vi "ecg_ncs_v2b.vi"() -> ()   [LabVIEW 2016]
uses:
  <instrlib>/niUSRP/niUSRP Timestamp.ctl
  C:/Program Files/National Instruments/LabVIEW 2016/examples/Instrument IO/Serial/support/Serial - Settings.ctl
  <vilib>/Analysis/coordinate.llb/Wrap Angle (array).vi
  <instrlib>/niUSRP/niUSRP Configure Time Start Trigger.vi
  <vilib>/Instr/_visa.llb/VISA Configure Serial Port (Instr).vi
  <vilib>/Analysis/3filter.llb/Butterworth Filter (DBL).vi
  <instrlib>/niUSRP/niUSRP Write Tx Data (2D CDB).vi
  <instrlib>/niUSRP/niUSRP Fetch Rx Data (2D CDB).vi
  <vilib>/measure/NI_MABase.lvlib
  <vilib>/Analysis/NI_AALBase.lvlib
  <vilib>/Analysis/NI_AALPro.lvlib
  <vilib>/Analysis/NI_AAL_Angle.lvlib
panel:
  out "Array":cdb[][](array[numeric])
  out "size(s) 4":i32[](array[numeric])
  out "timed out?":bool
  out "#sample":i32
  in  "timeout in ms (-1) 2":i32=-1
  in  "timeout in ms (-1)":i32=-1
  out "size(s) 3":i32
  out "size(s) 2":i32=10
  out "Serial Settings: \n#Bytes at Serial Port":u32
  in  "Stop":bool
  out "Poor Sensor Quality: \nSensor off":bool=TRUE
  out "Poor Sensor Quality: \nSensor on":bool
  out "Heart Rate 2":u16[](array[numeric])=[73]
  out "Stop Loop":bool
  out "Loop index":i32=16
  out "size(s)":i32=123
  in  "Read Count":u32=800
  out "return count":u32
  in  "Serial Settings":T1={"baud rate"=57600, "data bits"=8, "parity"=enum."None", "stop bits"=10, "flow control"=0} {"flow control" items=["None"=0, "XON/XOFF"=1, "RTS/CTS"=2, "DTR/DSR"=4]; "stop bits" items=["1.0"=10, "1.5"=15, "2.0"=20]; "data bits" min=5 max=8 step=1; "baud rate" items=["75"=75, "110"=110, "134"=134, "150"=150, "300"=300, "600"=600, "1200"=1200, "1800"=1800, "2400"=2400, "4800"=4800, "7200"=7200, "9600"=9600, "14400"=14400, "19200"=19200, "28800"=28800, "38400"=38400, "56000"=56000, "57600"=57600, "115200"=115200, "128000"=128000, "230400"=230400]}
  in  "VISA resource name":refnum<visa-resource-name>="bmd101"
  in  "?":enum32{"ECG", "Heart Rate"}(tab)
  out "?":i16(graph)=131
  out "?":u8[](graph)=[73]
  in  "File Name":string="Test"
  in  "order1":i32=5
  in  "Path":path=path "D:/Research/SummerFall17Spring18/CnC/NCS/EcgNcsCorrelation"
  in  "Low-Pass Freq":dbl=200.0 format="%#_13g"
  in  "Sampling Rate":i32=500
  out "Gain":dbl=-15.0
  out "Bandwidth":dbl=56000000.0
  out "Coerced Carrier Frequency":dbl=2000000000.0 format="%#.17g"
  out "Coerced Tx IQ rate":dbl=1000000.0
  out "Coerced Rx IQ rate":dbl=1000000.0
  out "error IO":errorcluster={"status"=FALSE, "code"=-1074118647, "source"=""}
  in  "Rx Number of Samples":i32=20000
  in  "Tab Control 2":enum32{"NI-294x/295x", "NI-2900/2901"}(tab)=enum."NI-2900/2901"
  in  "channel 0 carrier\n frequency [Hz]":dbl=2000000000.0 format="%#_6p"
  in  "Rx carrier frequency [Hz]":dbl=2000000000.0 format="%#_6p"
  in  "Tx carrier frequency [Hz]":dbl=1000000000.0 format="%#_6p"
  in  "Start Trigger Time":T2={"whole seconds"=1, "fractional seconds"=0.0}
  out "Tx Active Antenna":string="TX1"
  in  "Tab Control":T3(tab)
  out "NCS tag Amp":dbl[](graph)=[0.012547740464413999, 0.012546996275393813, 0.012546251124152991, 0.012545505011287303, 0.012544757937393139, 0.012544009903067494, 0.012543260908907984, 0.012542510955512811, 0.012541760043480784, 0.012541008173411305]
  out "NCS tag Phase":dbl[](graph)=[-1.392700873477184e-06, -1.383717662048323e-06, -1.3747392404395601e-06, -1.365765619105003e-06, -1.3567968084830664e-06, -1.3478328189964664e-06, -1.3388736610522184e-06, -1.3299193450416306e-06, -1.3209698813403015e-06, -1.3120252803081151e-06]
  out "IQ":dbl[][](graph)=[[-0.008331551052877154], [0.0]]
  out "Tag Amp":dbl[](graph)=[0.008331551052877154]
  out "Tag Phase":dbl[](graph)=[337.4998459209021]
  out "Tx Waveform Graph":waveform(dbl)[](graph)
  in  "Channel 0\nTone Amplitude":dbl=0.707 step=0.05 format="%#.6g"
  in  "Channel 0 \nTone Frequency":dbl=5000.0 format="%#_6p"
  in  "Waveform Size":dbl=1000.0
  in  "Rx Active Antenna":string="RX2"
  in  "Device Name":refnum<k15>="MyB200"
  in  "Tx Gain":dbl=28.0 format="%#_6f"
  in  "Tx IQ Rate":dbl=1000000.0 format="%#_6p"
  in  "Rx Gain":dbl=32.0 format="%#_6f"
  in  "Rx IQ Rate":dbl=1000000.0 format="%#_6p"
  # "Rx Settings"
  # "Tx Settings"
  # "Note that on the NI-2900 and NI-2901, both Rx channels share an LO and both Tx channels share an LO. However, on the NI-294x/295x devices, Rx and Tx of channel 0 share an LO and Rx and Tx of channel 1 share an LO."
  # "This Tx graph should always have end and start tied up since this is being sent in a loop continuously. Otherwise phase jumps will be noticed."
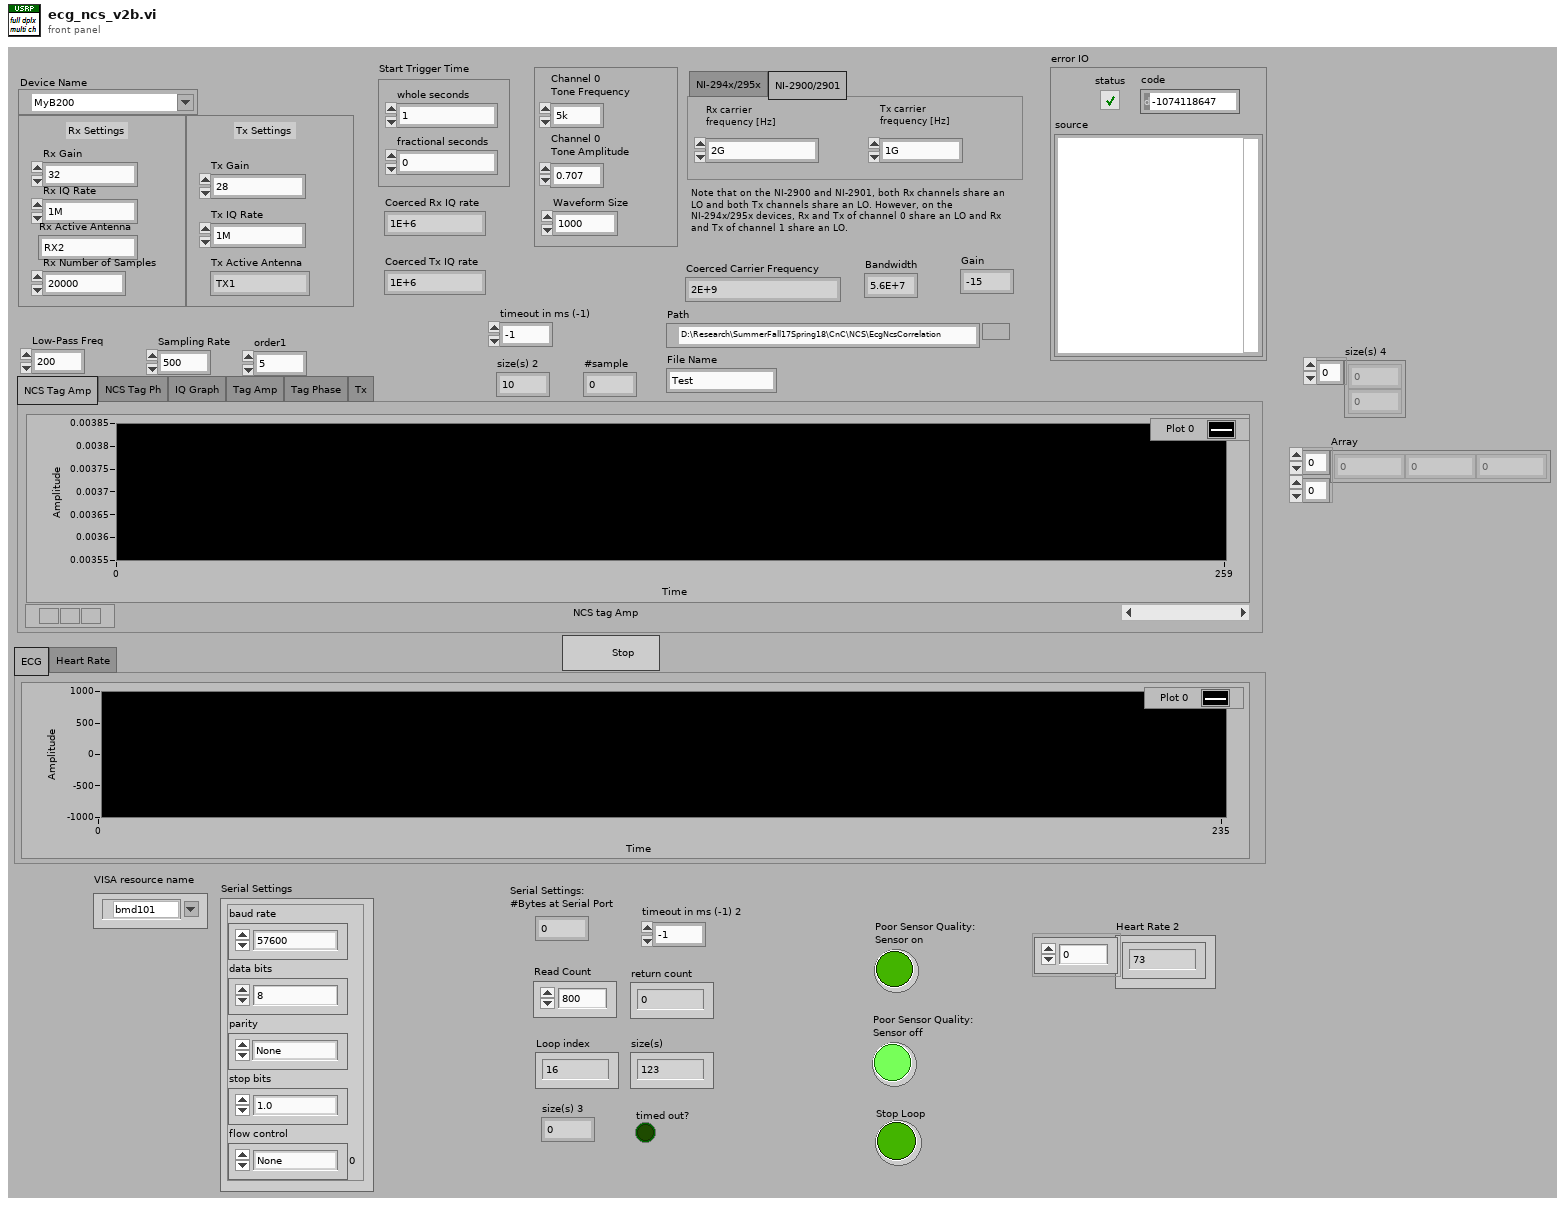
[diagram p1: front panel]
types:
  T1 = typedef "Serial - Settings.ctl" = cluster{"baud rate":u32, "data bits":u16, "parity":enum16{"None", "Odd", "Even", "Mark", "Space"}, "stop bits":u16, "flow control":u16}
  T2 = typedef "niUSRP Timestamp.ctl" = cluster{"whole seconds":u64, "fractional seconds":dbl}
  T3 = enum32{"NCS Tag Amp", "NCS Tag Ph", "IQ Graph", "Tag Amp", "Tag Phase", "Tx"}
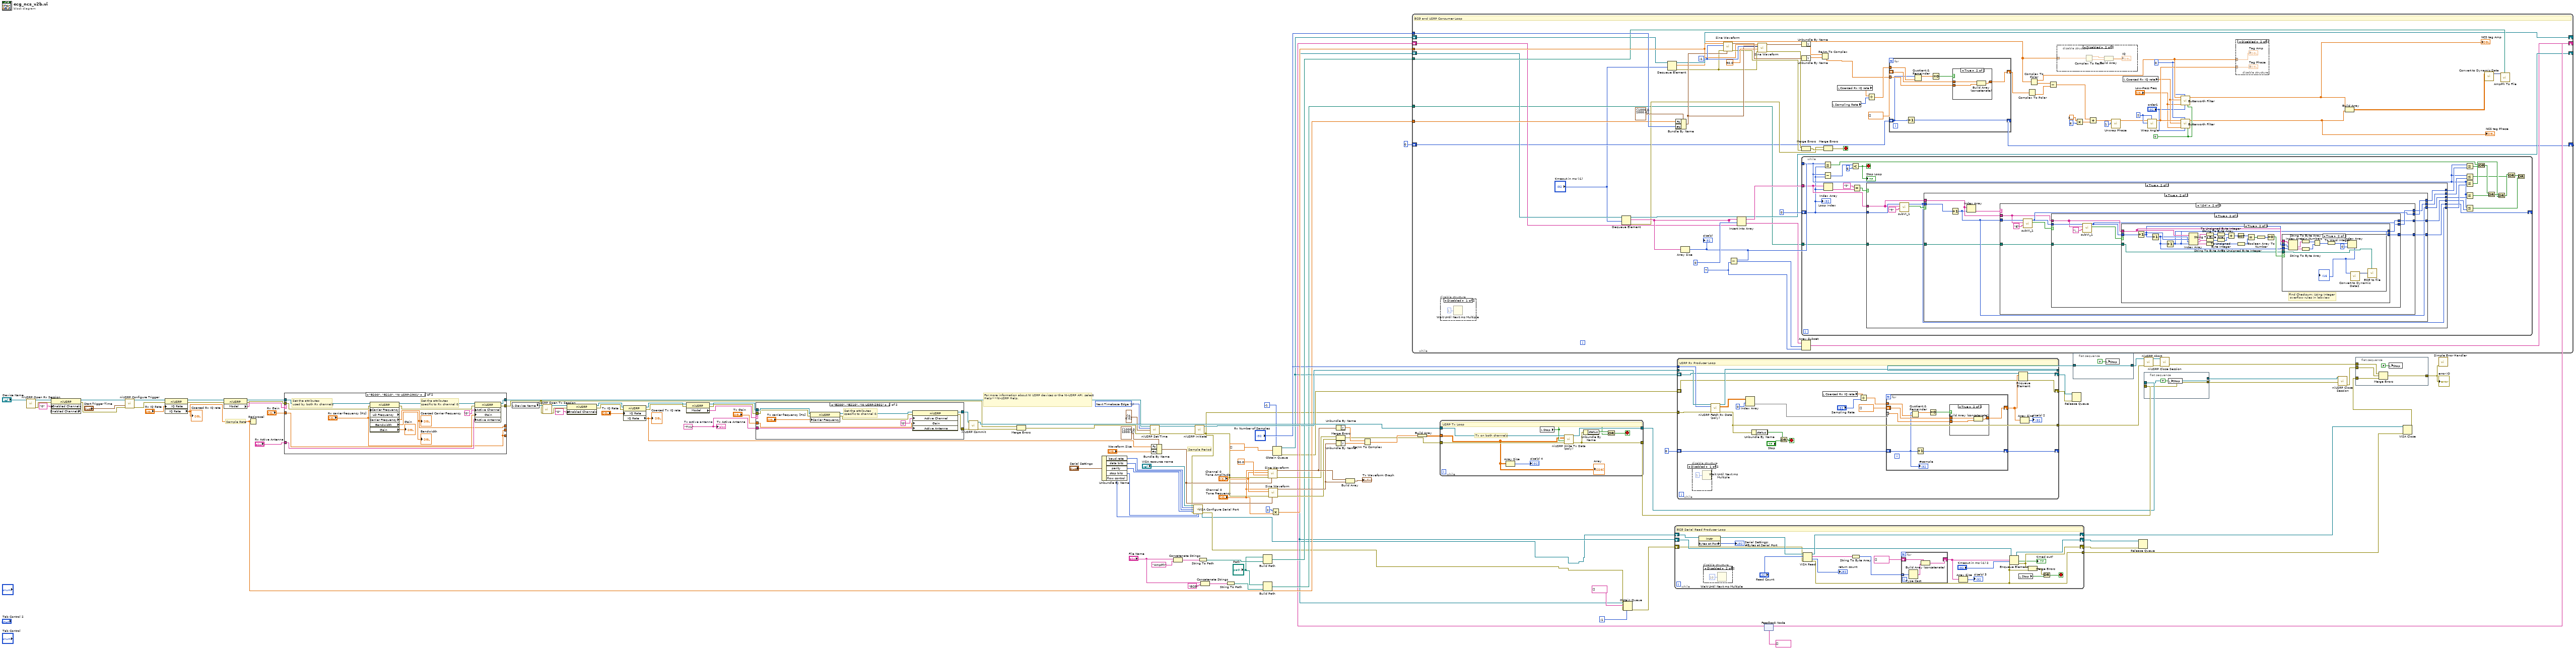
[diagram p0: block diagram]
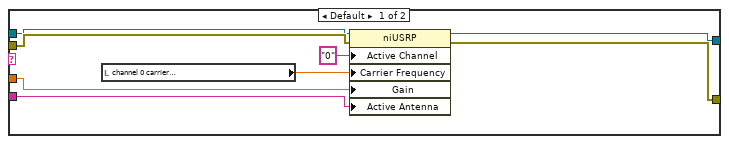
[diagram p5: hidden frame]
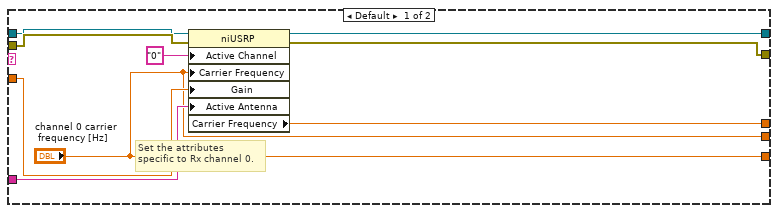
[diagram p6: hidden frame]
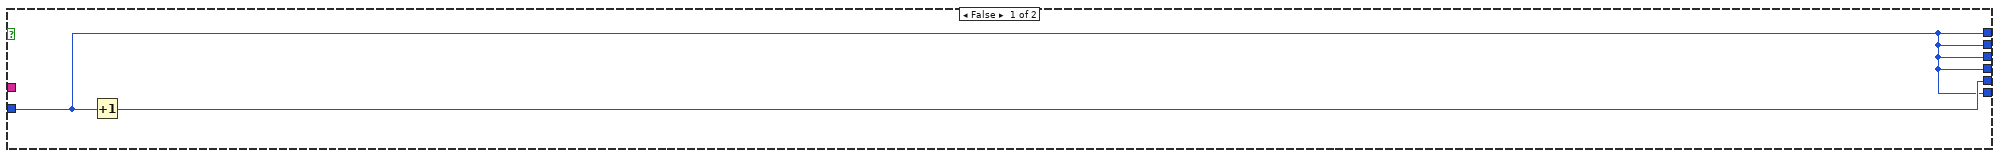
[diagram p9: hidden frame]
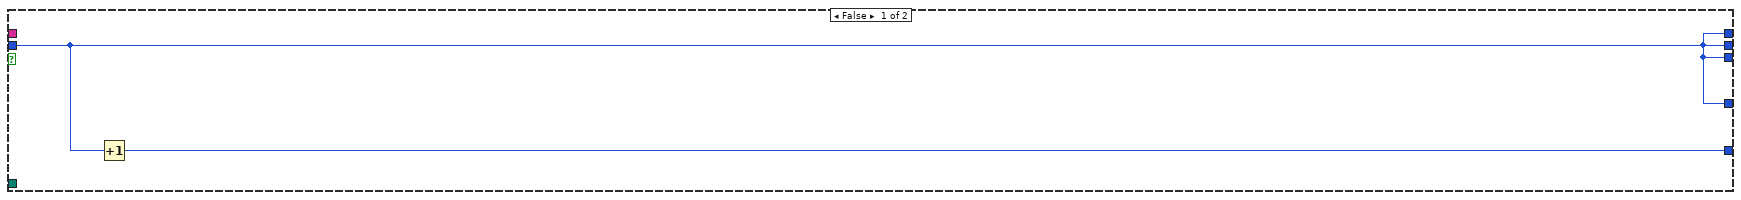
[diagram p10: hidden frame]
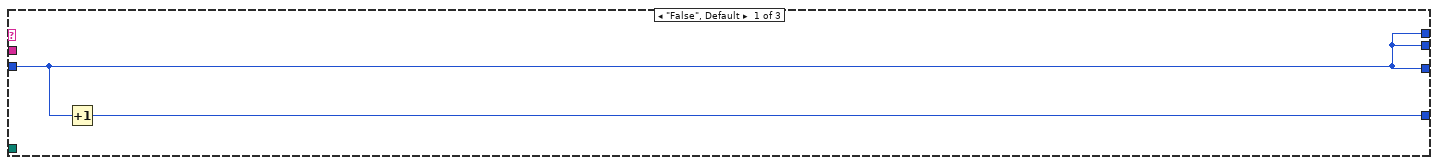
[diagram p11: hidden frame]
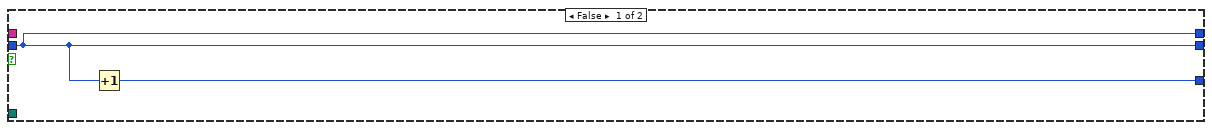
[diagram p12: hidden frame]
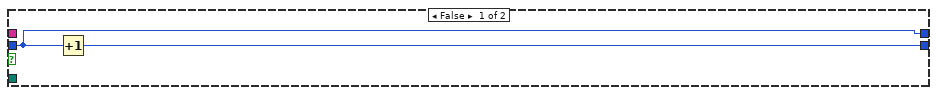
[diagram p13: hidden frame]
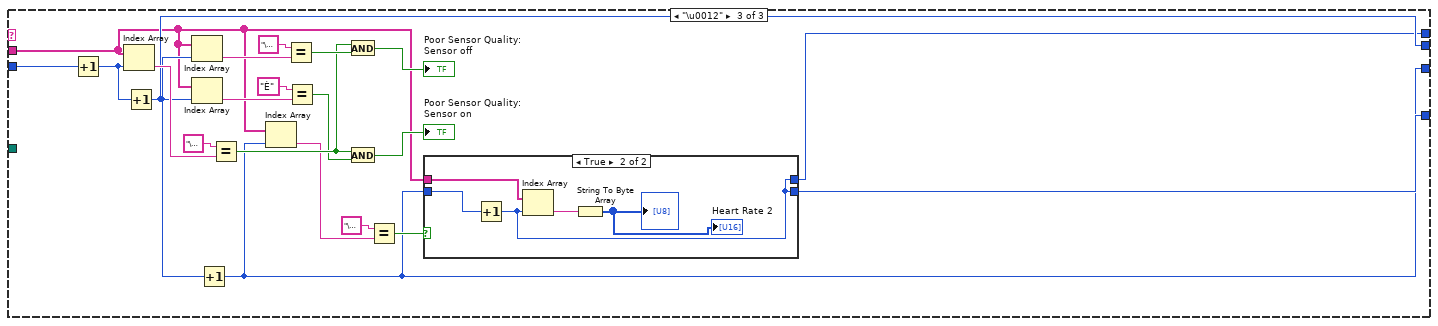
[diagram p15: hidden frame]
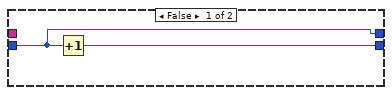
[diagram p16: hidden frame]
diagram:
  w91 = 1 items=["Now", "Next Timebase Edge"] ("apply timestamp")
  w60 = "TX1"  # Tx active antenna
  # "Sample Rate"
  # "Sample Period"
  # "For more information about NI USRP devices or the NI-USRP API, select Help>>NI-USRP Help."
  n1 = call <instrlib>:"niUSRP Open Rx Session.vi"("device names"="Device Name") -> ("session handle out"=w90:refnum<k15>, "error out"=w89:errorcluster)  [unwired: 13 in]
  n2 = property class="niUSRP" props=["Enabled Channels", "Enabled Channels"](reference=w90, error in=w89, "Enabled Channels"="0" ("Configuration:Enabled Channels")) -> (reference out=w88:refnum<k15>, error out=w87:errorcluster)  [unwired: 1 out]
  n3 = call-poly <instrlib>:"niUSRP Configure Trigger.vi"("session handle"=w88, "start trigger time"="Start Trigger Time", "error in (no error)"=w87) -> ("session handle out"=w84:refnum<k15>, "error out"=w83:errorcluster)  [unwired: 11 in]
  n4 = property class="niUSRP"(reference=w84, error in=w83, "IQ Rate"="Rx IQ Rate") -> (reference out=w80:refnum<k15>, error out=w81:errorcluster, "IQ Rate"=w19:dbl)
  "Coerced Rx IQ rate" <- w19
  n5 = property class="niUSRP"(reference=w80, error in=w81) -> (reference out=w75:refnum<k15>, error out=w76:errorcluster, "Model"=w77:string)
  n6 = Reciprocal(x=w19) -> ()  [unwired: 1 out]
  n7 = case shown="\"B200\", \"B210\", \"NI USRP-2901\"" w77 {
    tunnel: w76 -> [w124 w134]
    tunnel: w75 -> [w123 w135]
    tunnel: [w120 w131] -> w79
    tunnel: [w119 w130] -> w78
    tunnel: "Rx Gain" -> [w122 w137]
    tunnel: "Rx Active Antenna" -> [w121 w136]
    tunnel: [w117 w126] -> _
    tunnel: ["channel 0 carrier\n frequency [Hz]" "Rx carrier frequency [Hz]"] -> _
    tunnel: ["channel 0 carrier\n frequency [Hz]" "Rx carrier frequency [Hz]"] -> _
    frame Default {
      # "Set the attributes \nspecific to Rx channel 0."
      n8 = property class="niUSRP"(reference=w123, error in=w124, "Active Channel"="0", "Carrier Frequency"="channel 0 carrier\n frequency [Hz]", "Gain"=w122, "Active Antenna"=w121) -> (reference out=w120:refnum<k15>, error out=w119:errorcluster, "Carrier Frequency"=w117:dbl)
    }
    frame "B200", "B210", "NI USRP-2901" {
      # "Set the attributes \nused by both Rx channels"
      # "Set the attributes \nspecific to Rx channel 0."
      n9 = property class="niUSRP" props=["Carrier Frequency", "LO Frequency", "Carrier Frequency", "Bandwidth", "Gain"](reference=w135, error in=w134, "Carrier Frequency"="Rx carrier frequency [Hz]") -> (reference out=w133:refnum<k15>, error out=w132:errorcluster, "Carrier Frequency"=w126:dbl, "Bandwidth"=→"Bandwidth":dbl, "Gain"=→"Gain":dbl)  [unwired: 1 out]
      "Coerced Carrier Frequency" <- w126
      n10 = property class="niUSRP"(reference=w133, error in=w132, "Active Channel"="0", "Gain"=w137, "Active Antenna"=w136) -> (reference out=w131:refnum<k15>, error out=w130:errorcluster)
    }
  }
  n11 = local read "Device Name"() -> (w111:refnum<k15>)
  n12 = call <instrlib>:"niUSRP Open Tx Session.vi"("device names"=w111, "error in (no error)"=w78) -> ("session handle out"=w86:refnum<k15>, "error out"=w85:errorcluster)  [unwired: 12 in]
  n13 = property class="niUSRP"(reference=w86, error in=w85, "Enabled Channels"="0" ("Configuration:Enabled Channels")) -> (reference out=w72:refnum<k15>, error out=w71:errorcluster)
  n14 = property class="niUSRP"(reference=w72, error in=w71, "IQ Rate"="Tx IQ Rate") -> (reference out=w66:refnum<k15>, error out=w67:errorcluster, "IQ Rate"=w64:dbl)
  "Coerced Tx IQ rate" <- w64
  n15 = property class="niUSRP"(reference=w66, error in=w67) -> (reference out=w68:refnum<k15>, error out=w69:errorcluster, "Model"=w65:string)
  n16 = case shown="\"B200\", \"B210\", \"NI USRP-2901\"" w65 {
    tunnel: "Tx Gain" -> [w146 w156]
    tunnel: w60 -> [w144 w154]
    tunnel: [w140 w148] -> w62
    tunnel: [w139 w147] -> w63
    tunnel: w69 -> [w143 w150]
    tunnel: w68 -> [w142 w153]
    frame Default {
      n17 = local read "channel 0 carrier\n frequency [Hz]"() -> (w141:dbl)
      n18 = property class="niUSRP"(reference=w142, error in=w143, "Active Channel"="0", "Carrier Frequency"=w141, "Gain"=w146, "Active Antenna"=w144) -> (reference out=w140:refnum<k15>, error out=w139:errorcluster)
    }
    frame "B200", "B210", "NI USRP-2901" {
      # "Set the attributes \nspecific to channel 0."
      n19 = property class="niUSRP"(reference=w153, error in=w150, "Carrier Frequency"="Tx carrier frequency [Hz]") -> (reference out=w152:refnum<k15>, error out=w151:errorcluster)
      n20 = property class="niUSRP"(reference=w152, error in=w151, "Active Channel"="0", "Gain"=w156, "Active Antenna"=w154) -> (reference out=w148:refnum<k15>, error out=w147:errorcluster)
    }
  }
  n21 = call <instrlib>:"niUSRP Commit.vi"("session handle"=w62, "error in (no error)"=w63) -> ("session handle out"=w113:refnum<k15>, "error out"=w114:errorcluster)  [unwired: 12 in]
  n22 = Merge Errors(w78, w114) -> (w93:errorcluster)
  n23 = Unbundle By Name("Serial Settings") -> ("baud rate"=w26:u32, "data bits"=w27:u16, "parity"=w28:enum16{"None", "Odd", "Even", "Mark", "Space"}, "stop bits"=w29:u16, "flow control"=w30:u16)
  n24 = call <instrlib>:"niUSRP Set Time.vi"("session handle"=w79, "apply timestamp"=w91, "timestamp"=T2 {"whole seconds"=0, "fractional seconds"=0.0}, "error in (no error)"=w93) -> ("session handle out"=w95:refnum<k15>, "error out"=w94:errorcluster)  [unwired: 10 in]
  n25 = Bundle By Name(cluster=cluster{"Fs":dbl, "#s":dbl} {"Fs"=1000.0, "#s"=1000.0} ("sampling info"), "Fs"=w64, "#s"="Waveform Size") -> (w97:cluster{"Fs":dbl, "#s":dbl})
  n26 = Concatenate Strings("File Name", "AmpPh") -> (w44:string)
  n27 = call <instrlib>:"niUSRP Initiate.vi"("session handle"=w95, "error in (no error)"=w94) -> ("session handle out"=w22:refnum<k15>, "error out"=w1:errorcluster)  [unwired: 12 in]
  n28 = call-poly "VISA Configure Serial Port"("VISA resource name"="VISA resource name", "baud rate (9600)"=w26, "data bits (8)"=w27, "parity (0:none)"=w28, "error in (no error)"=w1, "stop bits (10: 1 bit)"=w29, "flow control (0:none)"=w30) -> ("VISA resource name out"=w2:refnum<visa-resource-name>, "error out"=w3:errorcluster)  [unwired: 3 in, 4 out]
  n29 = String To Path(string=w44) -> (path=w43:path)
  n30 = Concatenate Strings("File Name", "ECG") -> (w38:string)
  n31 = String To Path(string=w38) -> (path=w37:path)
  n32 = Build Path(base path="Path", name or relative path=w43) -> (appended path=w46:path)
  n33 = Build Path(base path="Path", name or relative path=w37) -> (appended path=w14:path)
  n34 = call <vilib>:"Sine Waveform.vi"("sampling info"=w97, "error in (no error)"=w1, "phase"=90.0, "amplitude"="Channel 0\nTone Amplitude", "frequency"="Channel 0 \nTone Frequency") -> ("error out"=w58:errorcluster, "signal out"=w105:waveform(dbl))  [unwired: 5 in]
  n35 = call <vilib>:"Sine Waveform.vi"("sampling info"=w97, "error in (no error)"=w1, "amplitude"="Channel 0\nTone Amplitude", "frequency"="Channel 0 \nTone Frequency") -> ("error out"=w59:errorcluster, "signal out"=w106:waveform(dbl))  [unwired: 6 in]
  n36 = Multiply(x=2, y="Channel 0 \nTone Frequency") -> (x*y=w47:dbl)
  n37 = Obtain Queue(max queue size (-1, unlimited)=-1, element data type=dbl[] []) -> (queue out=w16:refnum<queue>, error out=w5:errorcluster)  [unwired: 3 in, 1 out]
  n38 = Unbundle By Name(w105) -> ("Y"=w104:dbl[])
  n39 = Merge Errors(w58, w59) -> (w57:errorcluster)
  n40 = Unbundle By Name(w106) -> ("Y"=w103:dbl[])
  n41 = Build Array(w105, w106) -> (→"Tx Waveform Graph":waveform(dbl)[])
  n42 = Re/Im To Complex(1:w103, 2:w104) -> (0:w99:cdb[])
  n43 = Build Array(w99) -> (w98:cdb[][])
  n44 = while {
    tunnel: w113 -> [w165]
    tunnel: w57 -> [w164]
    tunnel: [w162] -> w56
    tunnel: [w160] -> w52
    tunnel: w98 -> [w158]
    stop <- w161 stop-if-true
    # "Tx on both channels"
    # "USRP Tx Loop"
    n45 = Array Size(array=w158) -> (size(s)=→"size(s) 4":i32[])
    n46 = local read "Stop"() -> (w159:bool)
    n47 = call-poly <instrlib>:"niUSRP Write Tx Data (poly).vi"("session handle"=w165, "data"=w158, "end of data?"=w159, "error in (no error)"=w164) -> ("session handle out"=w160:refnum<k15>, "error out"=w162:errorcluster)  [unwired: 10 in]
    n48 = Unbundle By Name(w162) -> ("status"=w163:bool)
    n49 = Compound Arithmetic op=OR(w163, w159) -> (w161:bool)
    "Array" <- w158
  }
  n50 = Obtain Queue(max queue size (-1, unlimited)=-1, element data type=string[] [], error in (no error)=w3) -> (queue out=w13:refnum<queue>, error out=w32:errorcluster)  [unwired: 2 in, 1 out]
  n51 = while {
    tunnel: [w166] -> w36
    shift-right: [w180] -> w34
    shift-left: w32 -> [w167]
    shift-right: [w181] -> w33
    shift-left: w13 -> [w182]
    shift-right: [w184] -> w35
    shift-left: w2 -> [w168]
    stop <- w186 stop-if-true
    # "ECG Serial Read Producer Loop"
    n52 = property class="Instr"(reference=w168) -> (reference out=w177:refnum<visa-resource-name>, "Bytes at Port"=→"Serial Settings: \n#Bytes at Serial Port":u32)  [unwired: 1 in, 1 out]
    n53 = disable-structure shown="Disabled" {
      frame Enabled {
      }
      frame Disabled {
        n54 = Wait Until Next ms Multiple(millisecond multiple=u32 10) -> ()  [unwired: 1 out]
      }
    }
    n55 = VISA Read(VISA resource name=w177, byte count="Read Count", error in (no error)=w167) -> (VISA resource name out=w184:refnum<visa-resource-name>, read buffer=w176:string, return count=→"return count":u32, error out=w166:errorcluster)
    n56 = String To Byte Array(string=w176) -> (unsigned byte array=w183:u8[])
    n57 = for {
      tunnel: w183 -> [w191] mode=indexing
      shift-right: [w188] -> w174
      shift-left: string[] [] -> [w189]
      n58 = Type Cast(x=w191) -> (*(type *) &x=w190:string)  [unwired: 1 in]
      n59 = Build Array (concatenate)(w189, w190) -> (w188:string[])
    }
    n60 = Array Size(array=w174) -> (size(s)=→"size(s) 3":i32)
    n61 = Enqueue Element(queue=w182, element=w174, timeout in ms (-1)="timeout in ms (-1) 2", error in (no error)=w166) -> (queue out=w181:refnum<queue>, timed out?=→"timed out?":bool, error out=w180:errorcluster)
    n62 = local read "Stop"() -> (w178:bool)
    n63 = Merge Errors(w180, w166) -> (w179:errorcluster)
    n64 = Or(x=w179, y=w178) -> (x .or. y?=w186:bool)
  }
  n65 = while {
    tunnel: w22 -> [w213]
    tunnel: [w212] -> w21
    tunnel: "Rx Number of Samples" -> [w211]
    tunnel: [w206] -> w15
    shift-right: [w208] -> w17
    shift-left: w16 -> [w209]
    shift-right: [w194] -> _
    shift-left: 0 -> [w195]
    tunnel: w1 -> [w207]
    shift-right: [w193] -> w4
    shift-left: w5 -> [w192]
    stop <- w210 stop-if-true
    # "USRP Rx Producer Loop"
    n66 = disable-structure shown="Disabled" {
      frame Disabled {
        n67 = Wait Until Next ms Multiple(millisecond multiple=u32 1 ("milliseconds to wait")) -> ()  [unwired: 1 out]
      }
      frame Enabled {
      }
    }
    n68 = call-poly <instrlib>:"niUSRP Fetch Rx Data (poly).vi"("session handle"=w213, "number of samples"=w211, "error in (no error)"=w207) -> ("session handle out"=w212:refnum<k15>, "data"=w204:cdb[][], "error out"=w206:errorcluster)  [unwired: 9 in, 1 out]
    n69 = Index Array(array=w204, index (row)=0 ("y")) -> (element=w198:cdb[])  [unwired: 1 in]
    n70 = Unbundle By Name(w206) -> ("status"=w214:bool)
    n71 = Or(x=w214, y="Stop") -> (x .or. y?=w210:bool)
    n72 = local read "Coerced Rx IQ rate"() -> (w202:dbl)
    n73 = Divide(x=w202, y="Sampling Rate") -> (x/y=w200:dbl)
    n74 = for {
      tunnel: w198 -> [w222] mode=indexing
      shift-right: [w220] -> w197
      shift-left: dbl[] [] -> [w221]
      tunnel: w200 -> [w217]
      shift-right: [w215] -> w194
      shift-left: w195 -> [w216]
      n75 = Quotient & Remainder(x=w216, y=w217) -> (x-y*floor(x/y)=w218:dbl)  [unwired: 1 out]
      n76 = Increment(x=w216) -> (x+1=w215:i32)
      n77 = Equal To 0?(x=w218) -> (x = 0?=w219:bool)
      n78 = case shown="True" w219 {
        tunnel: w222 -> [_ w226]
        tunnel: w221 -> [w223 w225]
        tunnel: [w223 w224] -> w220
        frame False {
        }
        frame True {
          n79 = Build Array (concatenate)(w225, w226) -> (w224:cdb[])
        }
      }
      "#sample" <- w216
    }
    n80 = Enqueue Element(queue=w209, element=w197, error in (no error)=w192) -> (queue out=w208:refnum<queue>, error out=w193:errorcluster)  [unwired: 1 in, 1 out]
    n81 = Array Size(array=w197) -> (size(s)=→"size(s) 2":i32)
  }
  n82 = feedback #1(string[] []) -> (w9:string[])
  n83 = while {
    tunnel: "Rx Number of Samples" -> [w288]
    tunnel: w19 -> [w280]
    tunnel: w47 -> [w281]
    tunnel: w46 -> [w279]
    shift-right: [w257] -> _
    shift-left: w16 -> [w258]
    tunnel: w14 -> [w234]
    shift-right: [w249] -> _
    shift-left: w13 -> [w250]
    shift-right: [w246] -> w12
    shift-left: w9 -> [w245]
    shift-right: [w229] -> _
    shift-left: 0 -> [w230]
    stop <- w248 stop-if-true
    w254 = 7
    w268 = 2 ("y")
    w261 = TRUE
    w263 = 0
    w286 = -1
    # "ECG and USRP Consumer Loop"
    n84 = disable-structure shown="Disabled" {
      frame Disabled {
        n85 = Wait Until Next ms Multiple(millisecond multiple=u32 1) -> ()  [unwired: 1 out]
      }
      frame Enabled {
      }
    }
    n86 = Dequeue Element(queue=w250, timeout in ms (-1)="timeout in ms (-1)") -> (queue out=w249:refnum<queue>, element=w247:string[], error out=w242:errorcluster)  [unwired: 1 in, 1 out]
    n87 = Dequeue Element(queue=w258, timeout in ms (-1)="timeout in ms (-1)") -> (queue out=w257:refnum<queue>, element=w241:dbl[], error out=w244:errorcluster)  [unwired: 1 in, 1 out]
    n88 = Bundle By Name(cluster=cluster{"Fs":dbl, "#s":dbl} {"Fs"=1000.0, "#s"=1000.0} ("sampling info"), "Fs"=w280, "#s"=w288) -> (w285:cluster{"Fs":dbl, "#s":dbl})
    n89 = Array Size(array=w247) -> (size(s)=w252:i32)
    "size(s)" <- w252
    n90 = call <vilib>:"Sine Waveform.vi"("sampling info"=w285, "error in (no error)"=w244, "amplitude"=w286, "frequency"=w281) -> ("error out"=w284:errorcluster, "signal out"=w289:waveform(dbl))  [unwired: 6 in]
    n91 = Subtract(x=w252, y=w254) -> (x-y=w253:i32)
    n92 = Insert Into Array(array=w247, index=0, new element=w245) -> (w255:string[])
    n93 = call <vilib>:"Sine Waveform.vi"("sampling info"=w285, "error in (no error)"=w244, "phase"=90.0, "amplitude"=w286, "frequency"=w281) -> ("error out"=w283:errorcluster, "signal out"=w282:waveform(dbl))  [unwired: 5 in]
    n94 = Unbundle By Name(w282) -> ("Y"=w277:dbl[])
    n95 = Unbundle By Name(w289) -> ("Y"=w276:dbl[])
    n96 = Merge Errors(w283, w284) -> (w243:errorcluster)
    n97 = while {
      tunnel: w255 -> [w325]
      shift-right: [w329] -> _
      shift-left: 0 -> [w308]
      tunnel: w252 -> [w309]
      tunnel: w234 -> [w304]
      stop <- w305 stop-if-true
      n98 = Less Or Equal?(x=w309, y=w308) -> (x <= y?=w310:bool)
      n99 = Subtract(x=w309, y=w308) -> (x-y=w307:i32)
      n100 = Index Array(array=w325, index=w308) -> (element=w328:string)
      n101 = Less?(x=w307, y=6) -> (x < y?=w305:bool)
      "Stop Loop" <- w305
      n102 = Equal?(x="ª", y=w328) -> (x = y?=w326:bool)
      n103 = case shown="True" w326 {
        tunnel: w308 -> [w330 w341]
        tunnel: [w331 w339] -> w329
        tunnel: w325 -> [_ w333]
        tunnel: [w330 w338] -> w324
        tunnel: [w330 w337] -> w322
        tunnel: [w330 w336] -> w319
        tunnel: [w330 w335] -> w316
        tunnel: [w330 w334] -> w313
        tunnel: w304 -> [_ w332]
        frame False {
          n104 = Increment(x=w330) -> (x+1=w331:i32)
        }
        frame True {
          n105 = call "subVI_1.vi"("String"="ª", "Array"=w333, "Numeric in"=w341) -> ("Boolean"=w340:bool, "Numeric out"=w338:i32)  [unwired: 7 in]
          n106 = case shown="True" w340 {
            tunnel: w338 -> [w343 w347]
            tunnel: [w344 w353] -> w339
            tunnel: w333 -> [_ w352]
            tunnel: [w343 w348] -> w337
            tunnel: [w343 w351] -> w336
            tunnel: [w343 w350] -> w335
            tunnel: [w343 w349] -> w334
            tunnel: w332 -> [_ w345]
            frame False {
              n107 = Increment(x=w343) -> (x+1=w344:i32)
            }
            frame True {
              n108 = Increment(x=w347) -> (x+1=w348:i32)
              n109 = Index Array(array=w352, index=w348) -> (element=w346:string)
              n110 = case shown="\"\\04\"" w346 {
                tunnel: w348 -> [w354 w361 w429]
                tunnel: [w355 w364 w411] -> w353
                tunnel: w352 -> [_ w357 w413]
                tunnel: [w354 w359 w415] -> w351
                tunnel: [w354 w363 w412] -> w350
                tunnel: [w354 w362 w410] -> w349
                tunnel: w345 -> [_ w356 _]
                frame "False", Default {
                  n111 = Increment(x=w354) -> (x+1=w355:i32)
                }
                frame "\u0004" {
                  n112 = call "subVI_1.vi"("String"="€", "Array"=w357, "Numeric in"=w361) -> ("Boolean"=w358:bool, "Numeric out"=w359:i32)  [unwired: 7 in]
                  n113 = case shown="True" w358 {
                    tunnel: w359 -> [w365 w372]
                    tunnel: [w366 w374] -> w364
                    tunnel: w357 -> [_ w371]
                    tunnel: [w365 w369] -> w363
                    tunnel: [w365 w373] -> w362
                    tunnel: w356 -> [_ w367]
                    frame False {
                      n114 = Increment(x=w365) -> (x+1=w366:i32)
                    }
                    frame True {
                      n115 = call "subVI_1.vi"("String"="\u0002", "Array"=w371, "Numeric in"=w372) -> ("Boolean"=w368:bool, "Numeric out"=w369:i32)  [unwired: 7 in]
                      n116 = case shown="True" w368 {
                        tunnel: w369 -> [w375 w381]
                        tunnel: [w376 w378] -> w374
                        tunnel: w371 -> [_ w382]
                        tunnel: [w375 w378] -> w373
                        tunnel: w367 -> [_ w377]
                        frame False {
                          n117 = Increment(x=w375) -> (x+1=w376:i32)
                        }
                        frame True {
                          # "Find Checksum: Using Integer\n overflow rules in labview"
                          n118 = Increment(x=w381) -> (x+1=w380:i32)
                          n119 = Increment(x=w380) -> (x+1=w379:i32)
                          n120 = Increment(x=w379) -> (x+1=w378:i32)
                          n121 = Index Array(array=w382, index #1=w380, index #2=w379, index #3=w378) -> (element #1=w396:string, element #2=w395:string, element #3=w389:string)
                          n122 = String To Byte Array(string=w396) -> (unsigned byte array=w394:u8[])
                          n123 = String To Byte Array(string=w395) -> (unsigned byte array=w393:u8[])
                          n124 = String To Byte Array(string=w389) -> (unsigned byte array=w388:u8[])
                          n125 = To Unsigned Byte Integer(number=w394) -> (unsigned 8bit integer=w392:u8[])
                          n126 = To Unsigned Byte Integer(number=w393) -> (unsigned 8bit integer=w391:u8[])
                          n127 = Add(x=w392, y=w391) -> (x+y=w390:u8[])
                          n128 = Not(x=w390) -> (.not. x?=w387:u8[])
                          n129 = To Unsigned Byte Integer(number=w388) -> (unsigned 8bit integer=w386:u8[])
                          n130 = Equal?(x=w387, y=w386) -> (x = y?=w385:bool[])
                          n131 = Boolean Array To Number(Boolean array=w385) -> (number=w384:u32)
                          n132 = Equal To 0?(x=w384) -> (x = 0?=w383:bool)
                          n133 = case shown="True" w383 {
                            tunnel: w382 -> [_ w409]
                            tunnel: w380 -> [_ w403]
                            tunnel: w379 -> [_ w402]
                            tunnel: w377 -> [_ w399]
                            frame False {
                            }
                            frame True {
                              n134 = Index Array(array=w409, index #1=w403, index #2=w402) -> (element #1=w408:string, element #2=w407:string)
                              n135 = String To Byte Array(string=w408) -> (unsigned byte array=w406:u8[])
                              n136 = String To Byte Array(string=w407) -> (unsigned byte array=w405:u8[])
                              n137 = Join Numbers(hi=w406, lo=w405) -> ((hi.lo)=w404:u16[])
                              n138 = To Word Integer(number=w404) -> (16bit integer=w401:i16[])
                              n139 = Index Array(array=w401, index=0) -> (element=w398:i16)
                              "?" <- w398
                              n140 = call "Convert to Dynamic Data2"("Double"=w398) -> ("Dynamic Data Type"=w397:dynamicdata)  [unwired: 3 in]
                              n141 = call "ECG to file"("Signals"=w397, "Filename"=w399) -> ()  [unwired: 15 in, 3 out]
                            }
                          }
                        }
                      }
                    }
                  }
                }
                frame "\u0012" {
                  n142 = Increment(x=w429) -> (x+1=w425:i32)
                  n143 = Index Array(array=w413, index=w425) -> (element=w428:string)
                  n144 = Increment(x=w425) -> (x+1=w415:i32)
                  n145 = Index Array(array=w413, index=w415) -> (element=w426:string)
                  n146 = Index Array(array=w413, index=w415) -> (element=w423:string)
                  n147 = Increment(x=w415) -> (x+1=w410:i32)
                  n148 = Equal?(x="\u0002", y=w428) -> (x = y?=w420:bool)
                  n149 = Index Array(array=w413, index=w410) -> (element=w416:string)
                  n150 = Equal?(x="\u0000", y=w426) -> (x = y?=w422:bool)
                  n151 = Equal?(x="È", y=w423) -> (x = y?=w419:bool)
                  n152 = And(x=w420, y=w422) -> (x .and. y?=→"Poor Sensor Quality: \nSensor off":bool)
                  n153 = And(x=w420, y=w419) -> (x .and. y?=→"Poor Sensor Quality: \nSensor on":bool)
                  n154 = Equal?(x="\u0003", y=w416) -> (x = y?=w414:bool)
                  n155 = case shown="True" w414 {
                    tunnel: w410 -> [w431 w437]
                    tunnel: w413 -> [_ w436]
                    tunnel: [w431 w435] -> w412
                    tunnel: [w432 w435] -> w411
                    frame False {
                      n156 = Increment(x=w431) -> (x+1=w432:i32)
                    }
                    frame True {
                      n157 = Increment(x=w437) -> (x+1=w435:i32)
                      n158 = Index Array(array=w436, index=w435) -> (element=w434:string)
                      n159 = String To Byte Array(string=w434) -> (unsigned byte array=→"Heart Rate 2" →"?":u8[])
                    }
                  }
                }
              }
            }
          }
        }
      }
      n160 = Less Or Equal?(x=w309, y=w319) -> (x <= y?=w317:bool)
      n161 = Less Or Equal?(x=w309, y=w316) -> (x <= y?=w314:bool)
      n162 = Less Or Equal?(x=w309, y=w324) -> (x <= y?=w323:bool)
      n163 = Less Or Equal?(x=w309, y=w322) -> (x <= y?=w320:bool)
      n164 = Less Or Equal?(x=w309, y=w313) -> (x <= y?=w311:bool)
      n165 = Or(x=w310, y=w323) -> (x .or. y?=w321:bool)
      n166 = Or(x=w321, y=w320) -> (x .or. y?=w318:bool)
      n167 = Or(x=w318, y=w317) -> (x .or. y?=w315:bool)
      n168 = Or(x=w315, y=w314) -> (x .or. y?=w312:bool)
      n169 = Or(x=w312, y=w311) -> ()  [unwired: 1 out]
      "Loop index" <- w308
    }
    n170 = Array Subset(array=w247, index=w253, length=w254) -> (w246:string[])
    n171 = Re/Im To Complex(1:w276, 2:w277) -> (0:w237:cdb[])
    n172 = Merge Errors(w242, w243) -> (w248:errorcluster)
    n173 = local read "Sampling Rate"() -> (w235:i32)
    n174 = local read "Coerced Rx IQ rate"() -> (w239:dbl)
    n175 = Divide(x=w239, y=w235) -> (x/y=w238:dbl)
    n176 = for {
      tunnel: w237 -> [w299] mode=indexing
      shift-right: [w297] -> w236
      shift-left: dbl[] [] -> [w298]
      tunnel: w238 -> [w294]
      shift-right: [w292] -> w229
      shift-left: w230 -> [w293]
      n177 = Increment(x=w293) -> (x+1=w292:i32)
      n178 = Quotient & Remainder(x=w293, y=w294) -> (x-y*floor(x/y)=w295:dbl)  [unwired: 1 out]
      n179 = Equal To 0?(x=w295) -> (x = 0?=w296:bool)
      n180 = case shown="True" w296 {
        tunnel: w299 -> [_ w303]
        tunnel: w298 -> [w300 w302]
        tunnel: [w300 w301] -> w297
        frame False {
        }
        frame True {
          n181 = Build Array (concatenate)(w302, w303) -> (w301:cdb[])
        }
      }
    }
    n182 = Complex To Polar(r * e^(i*theta)=w236) -> (theta=w271:dbl[])  [unwired: 1 out]
    n183 = Complex To Polar(r * e^(i*theta)=w241) -> (r=w278:dbl[], theta=w266:dbl[])
    n184 = Subtract(x=w266, y=w271) -> (x-y=w270:dbl[])
    n185 = disable-structure shown="Disabled" {
      disable-tunnel: w241 -> [_ w440]
      frame Enabled {
      }
      frame Disabled {
        n186 = Complex To Re/Im(x + iy=w440) -> (x=w443:dbl[], y=w442:dbl[])
        n187 = Build Array(w443, w442) -> (→"IQ":dbl[][])
      }
    }
    n188 = Multiply(x=3.141592653589793, y=6) -> (x*y=w272:dbl)
    n189 = Add(x=w270, y=w272) -> (x+y=w269:dbl[])
    n190 = call <vilib>:"Unwrap Phase.vi"("phase unit"=1 ("y"), "Phase"=w269) -> ("Unwrapped Phase"=w267:dbl[])  [unwired: 8 in, 1 out]
    n191 = local read "Coerced Rx IQ rate"() -> (w264:dbl)
    n192 = call-poly <vilib>:"Wrap Angle.vi"("angle units"=w268, "angle range"=w268, "Angle In"=w267) -> ("Angle Out"=w265:dbl[])  [unwired: 7 in, 1 out]
    n193 = call-poly <vilib>:"Butterworth Filter.vi"("init/cont (init:F)"=w261, "order"="order1", "filter type"=w263, "low cutoff freq: fl"="Low-Pass Freq", "sampling freq: fs"=w264, "X"=w278) -> ("Filtered X"=w233:dbl[])  [unwired: 2 in, 1 out]
    "NCS tag Amp" <- w233
    n194 = call-poly <vilib>:"Butterworth Filter.vi"("init/cont (init:F)"=w261, "order"="order1", "filter type"=w263, "low cutoff freq: fl"="Low-Pass Freq", "sampling freq: fs"=w264, "X"=w265) -> ("Filtered X"=w232:dbl[])  [unwired: 2 in, 1 out]
    "NCS tag Phase" <- w232
    n195 = disable-structure shown="Disabled" {
      disable-tunnel: w278 -> [_ w439]
      disable-tunnel: w265 -> [_ w438]
      frame Enabled {
      }
      frame Disabled {
        "Tag Amp" <- w439
        "Tag Phase" <- w438
      }
    }
    n196 = Build Array(w233, w232) -> (w231:dbl[][])
    n197 = call "Convert to Dynamic Data"("2D Array"=w231) -> ("Dynamic Data Type"=w259:dynamicdata)  [unwired: 3 in]
    n198 = call "AmpPh To File"("Signals"=w259, "Filename"=w279) -> ()  [unwired: 15 in, 3 out]
  }
  n199 = feedback-in #1(w12) -> ()
  n200 = Release Queue(queue=w17, error in (no error)=w4) -> ()  [unwired: 1 in, 3 out]
  n201 = flat-sequence {
    tunnel: [w444] -> w54
    tunnel: w21 -> [w444]
    frame #0 {
      n202 = local write "Stop"(TRUE ("STOP")) -> ()
    }
  }
  n203 = Release Queue(queue=w33, error in (no error)=w34) -> ()  [unwired: 1 in, 3 out]
  n204 = call <instrlib>:"niUSRP Abort.vi"("session handle"=w54, "error in (no error)"=w15) -> ("session handle out"=w110:refnum<k15>, "error out"=w109:errorcluster)  [unwired: 12 in]
  n205 = flat-sequence {
    tunnel: [w447] -> w55
    tunnel: w56 -> [w447]
    tunnel: [w446] -> w53
    tunnel: w52 -> [w446]
    frame #0 {
      n206 = local write "Stop"(TRUE ("STOP")) -> ()
    }
  }
  n207 = call <instrlib>:"niUSRP Close Session.vi"("session handle"=w110, "error in (no error)"=w109) -> ("error out"=w50:errorcluster)  [unwired: 13 in]
  n208 = call <instrlib>:"niUSRP Close Session.vi"("session handle"=w53, "error in (no error)"=w55) -> ("error out"=w51:errorcluster)  [unwired: 13 in]
  n209 = flat-sequence {
    tunnel: w51 -> [w452]
    tunnel: [w451] -> w42
    tunnel: w50 -> [w450]
    tunnel: w23 -> [w449]
    frame #0 {
      n210 = Merge Errors(w450, w452, w449) -> (w451:errorcluster)
      n211 = local write "Stop"(FALSE ("STOP")) -> ()
    }
  }
  n212 = VISA Close(VISA resource name=w35, error in (no error)=w36) -> (error out=w23:errorcluster)
  n213 = call <vilib>:"Simple Error Handler.vi"("error in (no error)"=w42) -> ()  [unwired: 1 in, 8 out]
  "Tx Active Antenna" <- w60
  "error IO" <- w42
